vi "Get Val DBL.vi"(8 "error in (no error)":errorcluster, 10 "Lookup String":string, 11 "PropertyObject in":refnum<class "PropertyObject.lvclass">) -> (0 "error out":errorcluster, 2 "Value":dbl, 3 "PropertyObject out":refnum<class "PropertyObject.lvclass">)   [LabVIEW 2020, in "TSnax.lvlib" / "PropertyObject.lvclass"]
uses:
  PropertyObject.lvclass
  PropertyObject.lvclass/PropertyObject.ctl
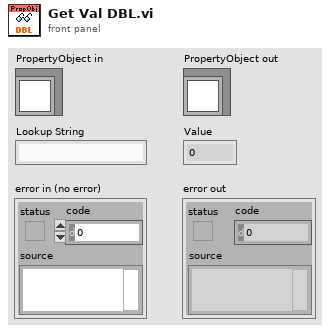
[diagram p1: front panel]
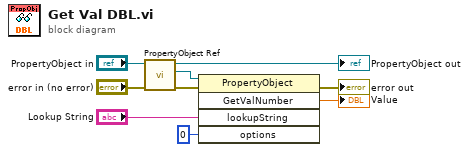
[diagram p0: block diagram]
diagram:
  n1 = call "PropertyObject Ref.vi"("error in (no error)"="error in (no error)", "PropertyObject in"="PropertyObject in") -> ("error out"=w4:errorcluster, "PropertyObject"=w7:refnum<k7>, "PropertyObject out"=→"PropertyObject out":refnum<class "PropertyObject.lvclass">)  [unwired: 7 in]
  n2 = invoke class="PropertyObject" method="GetValNumber"(reference=w7, error in=w4, "lookupString"="Lookup String", "options"=0) -> (error out=→"error out":errorcluster, "GetValNumber"=→"Value":dbl)  [unwired: 1 in, 3 out]
